vi "Prepare Data.vi"(0 "CS in":refnum<class "PCS.lvclass">, 2 "I0":T1 {"Current" min=0.0}, 3 "I1":T1 {"Current" min=0.0}, 4 "I2":T1 {"Current" min=0.0}, 5 "I3":T1 {"Current" min=0.0}, 7 "error in (no error)":errorcluster) -> (18 "Range bits":u32, 20 "CS out":refnum<class "PCS.lvclass">, 21 "V Out 0":dbl, 23 "V Out 1":dbl, 24 "V Out 2":dbl, 25 "V Out 3":dbl, 27 "error out":errorcluster)   [LabVIEW 2013, in "PCS.lvclass"]
uses:
  Lib.llb/PCS.lvclass
  Lib.llb/CS Data.ctl
  Lib.llb/QCS.lvclass
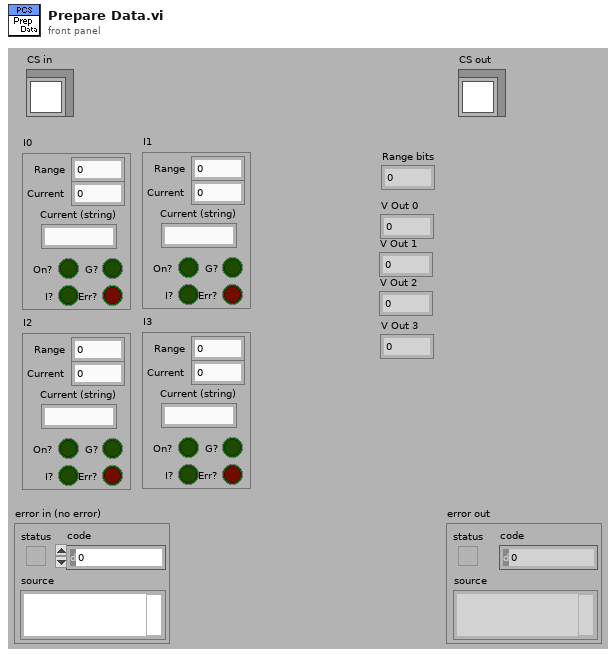
[diagram p1: front panel]
types:
  T1 = typedef "CS Data.ctl" = cluster{"Range":u8, "Current":dbl, "Current (string)":string, "On?":bool, "G?":bool, "I?":bool, "Err?":bool}
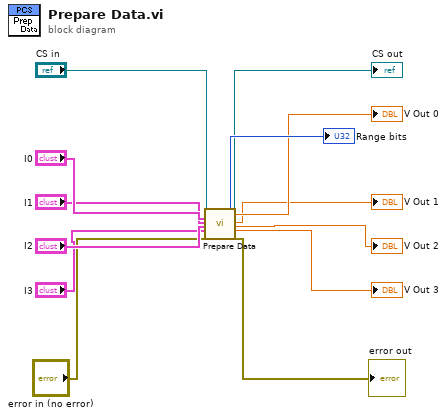
[diagram p0: block diagram]
diagram:
  n1 = call-parent "Prepare Data.vi"("CS in"="CS in", "I0"="I0", "I1"="I1", "I2"="I2", "I3"="I3", "error in (no error)"="error in (no error)") -> ("Range bits"=→"Range bits":u32, "CS out"=→"CS out":refnum<class "PCS.lvclass">, "V Out 0"=→"V Out 0":dbl, "V Out 1"=→"V Out 1":dbl, "V Out 2"=→"V Out 2":dbl, "V Out 3"=→"V Out 3":dbl, "error out"=→"error out":errorcluster)  [unwired: 15 in]
